vi "Initialize UUT States.vi"(8 "error in (no error)":errorcluster, 10 "Number of UUTs":u32, 11 "Application in":refnum<class "Application.lvclass">) -> (0 "error out":errorcluster, 3 "Application out":refnum<class "Application.lvclass">)   [LabVIEW 2017, in "Application.lvlib" / "Application.lvclass"]
doc: "Used by child classes to initialize all UUTs to a specified \"State\" when starting a test. This could be handled as a Parent Class only with the exception of Applications using custom \"State\" objects."
uses:
  Application.lvclass
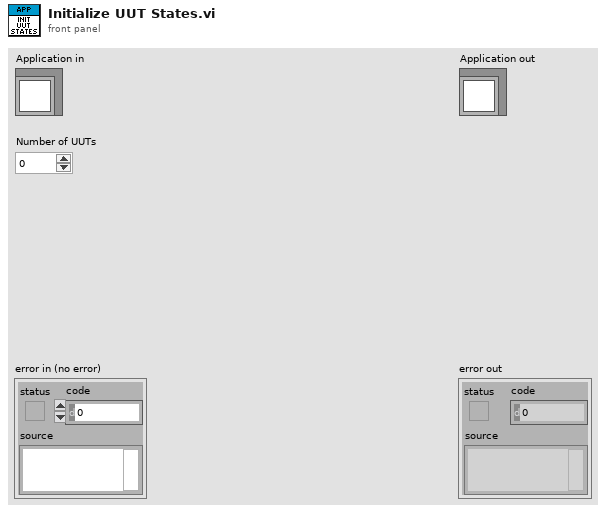
[diagram p1: front panel]
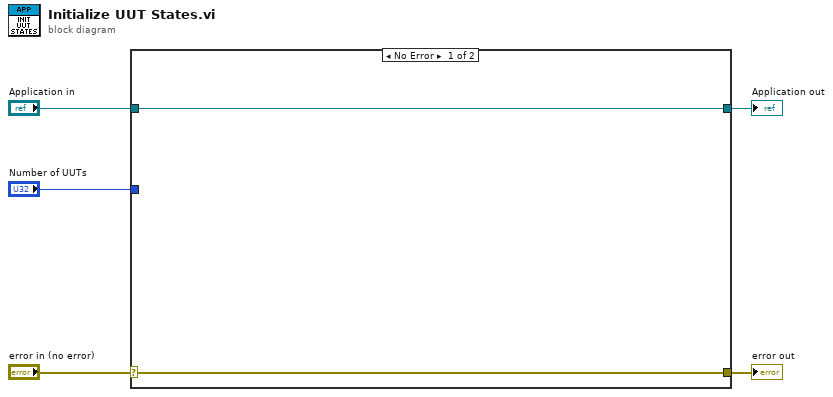
[diagram p0: block diagram]
diagram:
  n1 = case shown="No Error" "error in (no error)" {
    selector: "error in (no error)" -> [w6 w9]
    tunnel: [w6 w9] -> w4
    tunnel: [w7 w8] -> w2
    tunnel: "Application in" -> [w7 w8]
    tunnel: "Number of UUTs" -> [_ _]
    frame No Error {
    }
    frame Error {
    }
  }
  "error out" <- w4
  "Application out" <- w2
